vi "Read Keypad.vi"(8 "error in (no error)":errorcluster, 11 "Simulated User Console Actor in":refnum<class "Simulated User Console Actor.lvclass">) -> (0 "error out":errorcluster, 3 "Simulated User Console Actor out":refnum<class "Simulated User Console Actor.lvclass">)   [LabVIEW 2019, in "Simulated User Console Actor.lvlib" / "Simulated User Console Actor.lvclass"]
uses:
  Simulated User Console Actor.lvclass
  C:/Program Files (x86)/National Instruments/LabVIEW 2019/vi.lib/ActorFramework/Actor/Actor.lvclass
  <vilib>/ActorFramework/Actor/Actor.lvclass/Actor.ctl
  Simulated User Console Actor.lvclass/Simulated User Console Actor.ctl
  ATM Controller/ATM Controller Messages/Get Screen Number Msg/Set Current Record from Keypad Msg.lvclass/Set Current Record from Keypad Msg.ctl
  <vilib>/ActorFramework/Message Enqueuer/Message Enqueuer.lvclass/Message Enqueuer.ctl
  <vilib>/ActorFramework/Message Enqueuer/Enqueue.vi
  ATM Controller/ATM Controller Messages/Get Screen Number Msg/Set Current Record from Keypad Msg.lvclass
  C:/Program Files (x86)/National Instruments/LabVIEW 2019/vi.lib/ActorFramework/Message/Message.lvclass
  <vilib>/ActorFramework/Message Priority Queue/Priority Enqueue.vi
  <vilib>/ActorFramework/Actor/Actor.lvclass
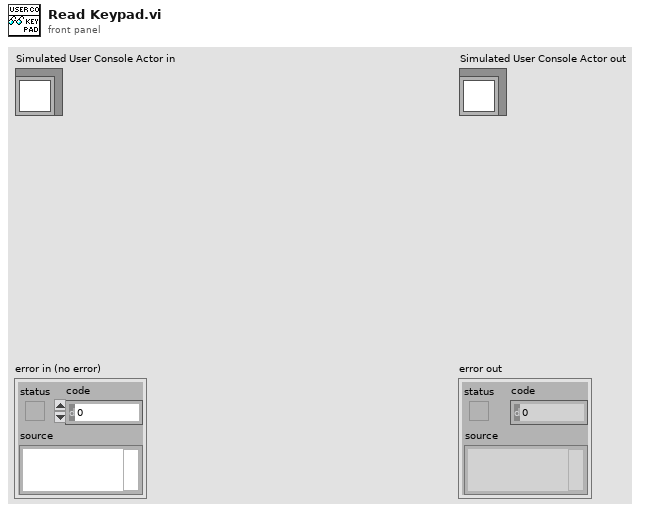
[diagram p1: front panel]
types:
  T1 = typedef "Simulated User Console Actor.lvlib/Simulated User Console Actor.lvclass/Keypad - Cluster.ctl" = cluster{"1":bool, "1 2":bool, "1 3":bool, "1 4":bool, "1 5":bool, "1 6":bool, "1 7":bool, "1 8":bool, "1 9":bool, "C":bool, "1 11":bool, "E":bool, "Screen":string}
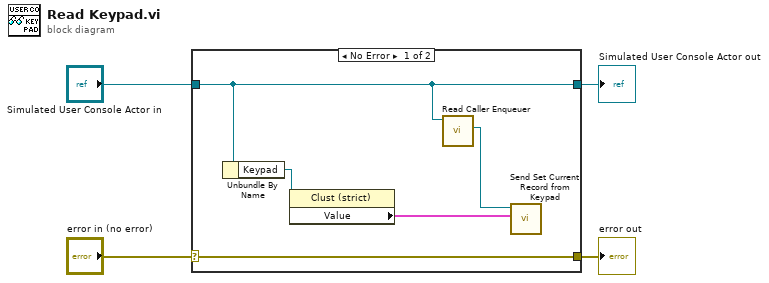
[diagram p0: block diagram]
diagram:
  n1 = case shown="No Error" "error in (no error)" {
    selector: "error in (no error)" -> [w9 w10]
    tunnel: [w9 w10] -> w3
    tunnel: [w7 w11] -> w1
    tunnel: "Simulated User Console Actor in" -> [w7 w11]
    frame No Error {
      n2 = Unbundle By Name(w7) -> ("Keypad"=w8:refnum<vi>)
      n3 = property class="Clust (strict)"(reference=w8) -> ("Value"=w5:T1)  [unwired: 1 in, 2 out]
      n4 = call <vilib>:"Read Caller Enqueuer.vi"("Actor"=w7) -> ("Caller Enqueuer"=w6:refnum<class "Message Enqueuer.lvclass">)  [unwired: 10 in]
      n5 = call "Send Set Current Record from Keypad.vi"("Keypad"=w5, "Message Enqueuer"=w6) -> ()  [unwired: 8 in, 2 out]
    }
    frame Error {
    }
  }
  "error out" <- w3
  "Simulated User Console Actor out" <- w1
